vi "case_stop_gcode.vi"(8 "error in (no error)":errorcluster, 11 "VI in":refnum<vi>) -> (0 "error out":errorcluster)   [LabVIEW 2020]
uses:
  f8656b25-7550-4219-b948-b6e4db7ec9c1.vi
  d6e257aa-2b27-4f83-b93a-ff047bc08312.vi
  59208b00-13f4-4418-8c60-f6e0eda57327.vi
  f1456ea9-36e7-4617-b532-97f947d7608e.vi
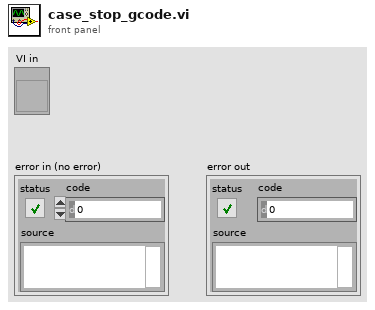
[diagram p1: front panel]
types:
  T1 = enum8{"Enabled", "Disabled", "Disabled and Grayed Out"}
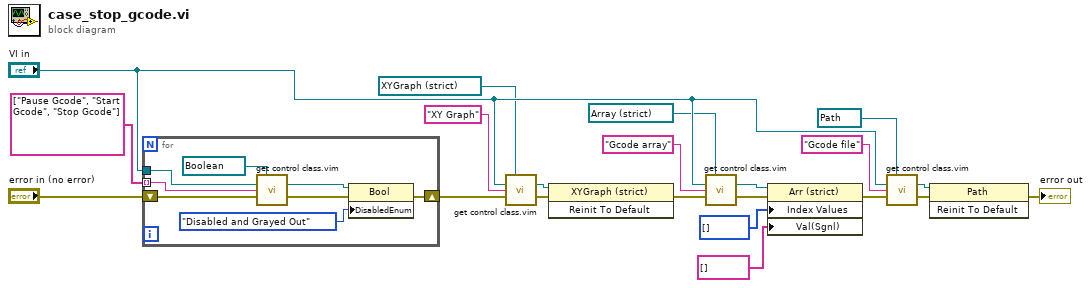
[diagram p0: block diagram]
diagram:
  n1 = for {
    tunnel: string[] ["Pause Gcode", "Start Gcode", "Stop Gcode"] -> [w29] mode=indexing
    tunnel: "VI in" -> [w25]
    shift-right: [w22] -> w16
    shift-left: "error in (no error)" -> [w23]
    n2 = call "get control class.vim"("Control class"=refnum<vi> refnum ("reference out"), "Main VI reference"=w25, "Label"=w29, "error in (no error)"=w23) -> ("Control out"=w28:refnum<vi>, "error out"=w27:errorcluster)  [unwired: 10 in]
    n3 = property on="Property Node" class="Bool"(reference=w28, error in=w27, "DisabledEnum"=T1."Disabled and Grayed Out" ("Disabled")) -> (error out=w22:errorcluster)  [unwired: 1 out]
  }
  n4 = call "get control class.vim"("Control class"=refnum<vi> refnum ("reference out"), "Main VI reference"="VI in", "Label"="XY Graph", "error in (no error)"=w16) -> ("Control out"=w9:refnum<vi>, "error out"=w10:errorcluster)  [unwired: 10 in]
  n5 = invoke on="Invoke Node" class="XYGraph (strict)" method="Reinit To Default"(reference=w9, error in=w10) -> (error out=w17:errorcluster)  [unwired: 1 in, 2 out]
  n6 = call "get control class.vim"("Control class"=refnum<vi> refnum ("reference out"), "Main VI reference"="VI in", "Label"="Gcode array", "error in (no error)"=w17) -> ("Control out"=w14:refnum<vi>, "error out"=w18:errorcluster)  [unwired: 10 in]
  n7 = property on="Property Node" class="Arr (strict)"(reference=w14, error in=w18, "Index Values"=u32[] [], "Val(Sgnl)"=string[] [] ("Value (Signaling)")) -> (error out=w19:errorcluster)  [unwired: 1 out]
  n8 = call "get control class.vim"("Control class"=refnum<vi> refnum ("reference out"), "Main VI reference"="VI in", "Label"="Gcode file", "error in (no error)"=w19) -> ("Control out"=w5:refnum<vi>, "error out"=w6:errorcluster)  [unwired: 10 in]
  n9 = invoke on="Invoke Node" class="Path" method="Reinit To Default"(reference=w5, error in=w6) -> (error out=→"error out":errorcluster)  [unwired: 1 in, 2 out]
